vi "Target Get Sensor Values.vi"(6 "Main Clock Line (s)":dbl) -> (0 "Vicon Log Trigger":dbl, 3 "Target Sensors":T1)   [LabVIEW 2018]
uses:
  Target Sensors.ctl
  COBRA-Libraries/Measurement and Filtering/COBRA Measurement and Filtering Library.lvlib
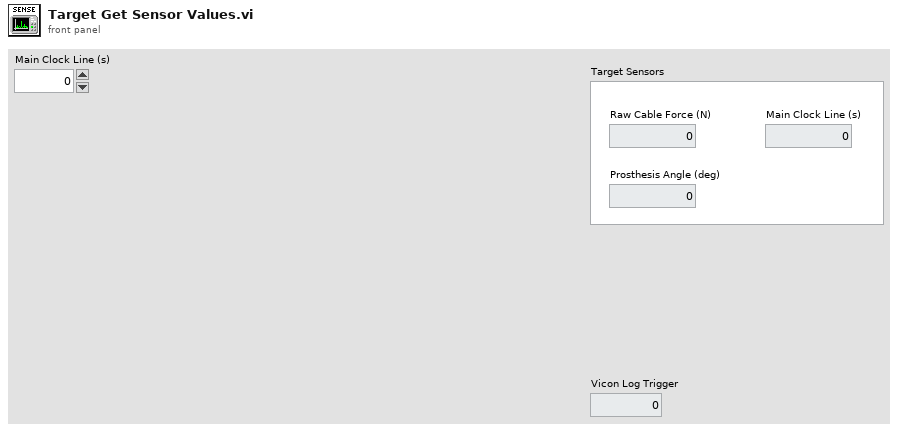
[diagram p1: front panel]
types:
  T1 = typedef "Target Sensors.ctl" = cluster{"Raw Cable Force (N)":dbl, "Prosthesis Angle (deg)":dbl, "Main Clock Line (s)":dbl}
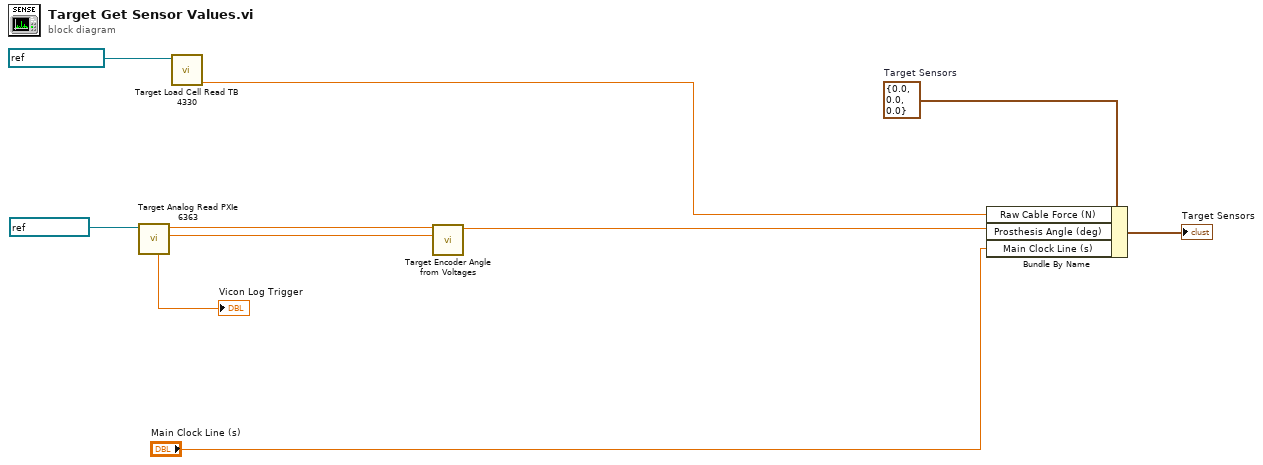
[diagram p0: block diagram]
diagram:
  w5 = T1 {"Raw Cable Force (N)"=0.0, "Prosthesis Angle (deg)"=0.0, "Main Clock Line (s)"=0.0}  # Target Sensors
  n1 = call "Target Analog Read PXIe 6363.vi"("task/channels in"=refnum<k21> "PXIe-6363") -> ("Encoder Voltage B"=w6:dbl, "Encoder Voltage A"=w7:dbl, "Vicon Log Trigger"=→"Vicon Log Trigger":dbl)  [unwired: 7 in, 1 out]
  n2 = call "Target Load Cell Read TB 4330.vi"("task/channels in"=refnum<k21> "Futek 844206") -> ("Cable Force (N)"=w2:dbl)  [unwired: 10 in]
  n3 = call "Target Encoder Angle from Voltages.vi"("Encoder Voltage B (V)"=w6, "Encoder Voltage A (V)"=w7) -> ("Encoder Angle (deg)"=w3:dbl)  [unwired: 9 in]
  n4 = Bundle By Name(cluster=w5, "Raw Cable Force (N)"=w2, "Prosthesis Angle (deg)"=w3, "Main Clock Line (s)"="Main Clock Line (s)") -> (→"Target Sensors":T1)
